vi "Load Plugin.vi"(8 "error in (no error)":errorcluster, 10 "Plugin":string) -> (0 "error out":errorcluster, 2 "Plugin":refnum<class "Plugin.lvclass">)   [LabVIEW 2020, in "Plugin Loader.lvclass"]
uses:
  Plugin Loader.lvclass
  Framework/Plugin/Plugin.lvclass
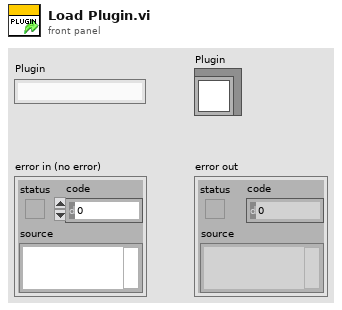
[diagram p1: front panel]
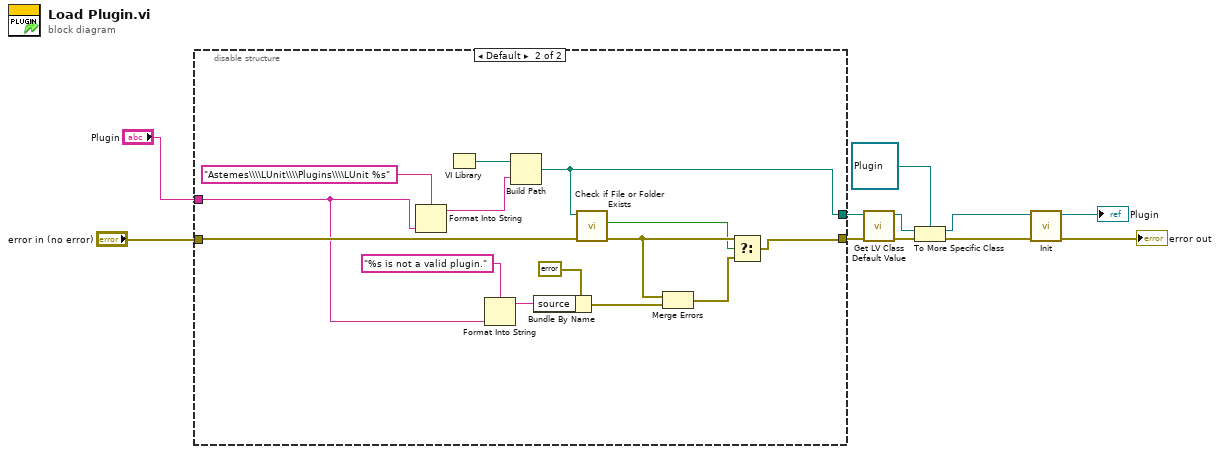
[diagram p0: block diagram]
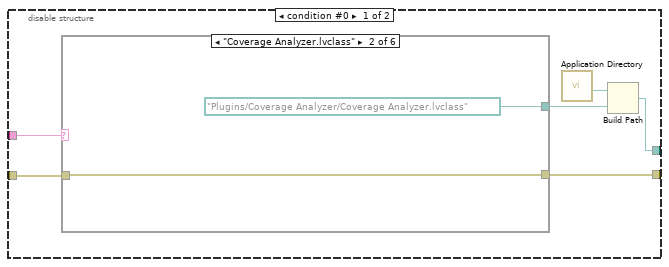
[diagram p2: hidden frame]
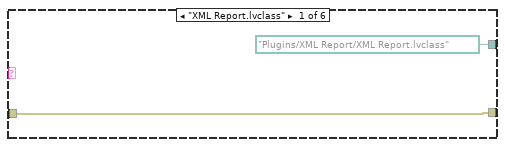
[diagram p3: hidden frame]
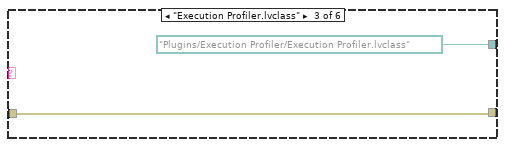
[diagram p4: hidden frame]
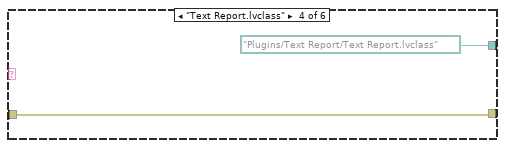
[diagram p5: hidden frame]
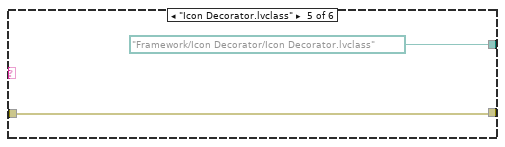
[diagram p6: hidden frame]
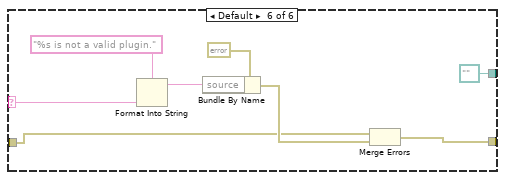
[diagram p7: hidden frame]
diagram:
  n1 = disable-structure shown="Default" {
    disable-tunnel: "Plugin" -> [w17 w41]
    disable-tunnel: "error in (no error)" -> [w16 w46]
    disable-tunnel: [w15 w39] -> w5
    disable-tunnel: [w12 w36] -> w1
    frame condition #0 {
      n2 = case shown="\"Coverage Analyzer.lvclass\"" w17 {
        selector: w17 -> [_ _ _ _ _ w31]
        tunnel: [w19 w21 w23 w25 w27 w29] -> w15
        tunnel: w16 -> [w19 w21 w23 w25 w27 w28]
        tunnel: [path "Plugins/XML Report/XML Report.lvclass" ("name or relative path") path "Plugins/Coverage Analyzer/Coverage Analyzer.lvclass" ("Relative Path from 1 to 2") path "Plugins/Execution Profiler/Execution Profiler.lvclass" ("Relative Path from 1 to 2") path "Plugins/Text Report/Text Report.lvclass" ("Relative Path from 1 to 2") path "Framework/Icon Decorator/Icon Decorator.lvclass" ("name or relative path") path "" ("name or relative path")] -> w13
        frame "XML Report.lvclass" {
        }
        frame "Coverage Analyzer.lvclass" {
        }
        frame "Execution Profiler.lvclass" {
        }
        frame "Text Report.lvclass" {
        }
        frame "Icon Decorator.lvclass" {
        }
        frame Default {
          n3 = Format Into String(format string="%s is not a valid plugin.", w31) -> (resulting string=w32:string)  [unwired: 2 in, 1 out]
          n4 = Bundle By Name(cluster=errorcluster {"status"=TRUE, "code"=7, "source"=""} ("error constant"), "source"=w32) -> (w34:errorcluster)
          n5 = Merge Errors(w28, w34) -> (w29:errorcluster)
        }
      }
      n6 = call <vilib>:"Application Directory.vi"() -> ("Application Directory"=w14:path)
      n7 = Build Path(base path=w14, name or relative path=w13) -> (appended path=w12:path)
    }
    frame condition #1 (active) {
      n8 = Format Into String(format string="Astemes\\\\LUnit\\\\Plugins\\\\LUnit %s" ("Relative Path from 1 to 2"), w41) -> (resulting string=w49:string)  [unwired: 2 in, 1 out]
      n9 = VI Library() -> (path=w48:path)
      n10 = Format Into String(format string="%s is not a valid plugin.", w41) -> (resulting string=w44:string)  [unwired: 2 in, 1 out]
      n11 = Build Path(base path=w48, name or relative path=w49) -> (appended path=w36:path)
      n12 = Bundle By Name(cluster=errorcluster {"status"=TRUE, "code"=7, "source"=""} ("error constant"), "source"=w44) -> (w45:errorcluster)
      n13 = call <vilib>:"Check if File or Folder Exists.vi"("error in (no error)"=w46, "path"=w36) -> ("error out"=w40:errorcluster, "file or folder exists?"=w38:bool)  [unwired: 7 in, 1 out]
      n14 = Merge Errors(w40, w45) -> (w37:errorcluster)
      n15 = Select(t=w40, s=w38, f=w37) -> (s? t:f=w39:errorcluster)
    }
  }
  n16 = call <vilib>:"Get LV Class Default Value.vi"("error in (no error)"=w5, "class path"=w1) -> ("error out"=w6:errorcluster, "object"=w7:refnum<class>)  [unwired: 8 in]
  n17 = To More Specific Class(target class=refnum<class "Plugin.lvclass"> refnum ("Plugin in"), reference=w7, error in=w6) -> (specific class reference=w3:refnum<class "Plugin.lvclass">, error out=w4:errorcluster)
  n18 = call-dynamic "Init.vi"("error in (no error)"=w4, "Plugin in"=w3) -> ("error out"=→"error out":errorcluster, "Plugin out"=→"Plugin":refnum<class "Plugin.lvclass">)  [unwired: 8 in]
